vi "Lissajou_Pattern_FOR.vi"() -> ()   [LabVIEW 2019]
panel:
  out "XY Graph":cluster{"X":dbl, "Y":dbl}[](graph)=[{"X"=0.9999996829318346, "Y"=0.0}, {"X"=0.9824361560225692, "Y"=0.12533323356430426}, {"X"=0.9300693384999064, "Y"=0.2486898871648548}, {"X"=0.8447543509816771, "Y"=0.368124552684678}, {"X"=0.7295135194338724, "Y"=0.4817536741017153}, {"X"=0.5884293077665393, "Y"=0.5877852522924731}, {"X"=0.42649969451448655, "Y"=0.6845471059286887}, {"X"=0.2494611169559819, "Y"=0.7705132427757893}, {"X"=0.06358525496231208, "Y"=0.8443279255020151}, {"X"=-0.1245431463883574, "Y"=0.9048270524660195}, {"X"=-0.3082595446881533, "Y"=0.9510565162951535}, {"X"=-0.4810556949368487, "Y"=0.9822872507286886}, {"X"=-0.6368102073656385, "Y"=0.9980267284282716}, {"X"=-0.7700054007214696, "Y"=0.9980267284282716}, {"X"=-0.8759227688762309, "Y"=0.9822872507286887}, {"X"=-0.9508101362587172, "Y"=0.9510565162951536}, {"X"=-0.9920145805448598, "Y"=0.9048270524660195}, {"X"=-0.9980764137536499, "Y"=0.844327925502015}, {"X"=-0.9687808924215839, "Y"=0.7705132427757895}, {"X"=-0.9051658249969167, "Y"=0.6845471059286888}, {"X"=-0.8094848069579887, "Y"=0.5877852522924732}, {"X"=-0.685127386069896, "Y"=0.4817536741017152}, {"X"=-0.5364989859650733, "Y"=0.36812455268467814}, {"X"=-0.36886484181482637, "Y"=0.24868988716485482}, {"X"=-0.18816347674844278, "Y"=0.1253332335643041}, {"X"=-0.000796326710733225, "Y"=1.2246467991473532e-16}, {"X"=0.18659903359770685, "Y"=-0.12533323356430384}, {"X"=0.36738403011337656, "Y"=-0.24868988716485457}, {"X"=0.535154264205682, "Y"=-0.3681245526846779}, {"X"=0.6839663916912916, "Y"=-0.4817536741017154}, {"X"=0.8085486687648371, "Y"=-0.587785252292473}, {"X"=0.9044877061514156, "Y"=-0.6845471059286887}, {"X"=0.9683848156219065, "Y"=-0.7705132427757894}, {"X"=0.9979764102178857, "Y"=-0.8443279255020153}, {"X"=0.9922141929481194, "Y"=-0.9048270524660198}, {"X"=0.9513022932321, "Y"=-0.9510565162951535}, {"X"=0.8766900355135938, "Y"=-0.9822872507286885}, {"X"=0.7710205962196693, "Y"=-0.9980267284282716}, {"X"=0.6380373679180319, "Y"=-0.9980267284282716}, {"X"=0.4824513477690753, "Y"=-0.9822872507286887}, {"X"=0.30977424810283877, "Y"=-0.9510565162951536}, {"X"=0.12612324126189484, "Y"=-0.9048270524660196}, {"X"=-0.06199574427856494, "Y"=-0.844327925502015}, {"X"=-0.24791849967043386, "Y"=-0.7705132427757896}, {"X"=-0.42505861861354033, "Y"=-0.684547105928689}, {"X"=-0.5871408240824221, "Y"=-0.5877852522924734}, {"X"=-0.7284232731434592, "Y"=-0.4817536741017153}, {"X"=-0.8439009646033401, "Y"=-0.36812455268467786}, {"X"=-0.9294830436715473, "Y"=-0.2486898871648545}, {"X"=-0.9821377225307751, "Y"=-0.12533323356430465}, {"X"=-0.9999996829318346, "Y"=-2.4492935982947064e-16}, {"X"=-0.9824361560225694, "Y"=0.1253332335643033}, {"X"=-0.9300693384999066, "Y"=0.24868988716485402}, {"X"=-0.844754350981678, "Y"=0.36812455268467736}, {"X"=-0.729513519433873, "Y"=0.4817536741017149}, {"X"=-0.5884293077665396, "Y"=0.5877852522924729}, {"X"=-0.4264996945144877, "Y"=0.6845471059286886}, {"X"=-0.24946111695598225, "Y"=0.7705132427757893}, {"X"=-0.06358525496231156, "Y"=0.8443279255020152}, {"X"=0.12454314638835703, "Y"=0.9048270524660194}, {"X"=0.3082595446881513, "Y"=0.9510565162951535}, {"X"=0.48105569493684763, "Y"=0.9822872507286886}, {"X"=0.6368102073656382, "Y"=0.9980267284282716}, {"X"=0.7700054007214688, "Y"=0.9980267284282716}, {"X"=0.8759227688762307, "Y"=0.9822872507286886}, {"X"=0.9508101362587175, "Y"=0.9510565162951536}, {"X"=0.9920145805448597, "Y"=0.9048270524660192}, {"X"=0.9980764137536499, "Y"=0.8443279255020151}, {"X"=0.9687808924215838, "Y"=0.7705132427757886}, {"X"=0.9051658249969168, "Y"=0.6845471059286884}, {"X"=0.809484806957989, "Y"=0.5877852522924734}, {"X"=0.6851273860698982, "Y"=0.4817536741017162}, {"X"=0.5364989859650751, "Y"=0.3681245526846796}, {"X"=0.36886484181482754, "Y"=0.2486898871648555}, {"X"=0.18816347674844575, "Y"=0.12533323356430567}, {"X"=0.0007963267107353688, "Y"=3.6739403974420594e-16}, {"X"=-0.1865990335977056, "Y"=-0.12533323356430318}, {"X"=-0.36738403011337295, "Y"=-0.24868988716485477}, {"X"=-0.535154264205681, "Y"=-0.36812455268467725}, {"X"=-0.6839663916912894, "Y"=-0.48175367410171555}, {"X"=-0.8085486687648374, "Y"=-0.5877852522924728}, {"X"=-0.904487706151415, "Y"=-0.6845471059286892}, {"X"=-0.9683848156219059, "Y"=-0.7705132427757891}, {"X"=-0.9979764102178857, "Y"=-0.8443279255020156}, {"X"=-0.9922141929481196, "Y"=-0.9048270524660197}, {"X"=-0.9513022932321007, "Y"=-0.9510565162951534}, {"X"=-0.8766900355135949, "Y"=-0.9822872507286885}, {"X"=-0.7710205962196708, "Y"=-0.9980267284282714}, {"X"=-0.6380373679180322, "Y"=-0.9980267284282716}, {"X"=-0.4824513477690771, "Y"=-0.9822872507286889}, {"X"=-0.3097742481028425, "Y"=-0.9510565162951538}, {"X"=-0.1261232412618952, "Y"=-0.90482705246602}, {"X"=0.061995744278562796, "Y"=-0.8443279255020152}, {"X"=0.24791849967043178, "Y"=-0.7705132427757898}, {"X"=0.42505861861354, "Y"=-0.6845471059286885}, {"X"=0.5871408240824219, "Y"=-0.5877852522924735}, {"X"=0.7284232731434602, "Y"=-0.48175367410171477}, {"X"=0.84390096460334, "Y"=-0.3681245526846781}, {"X"=0.9294830436715465, "Y"=-0.2486898871648556}, {"X"=0.9821377225307754, "Y"=-0.125333233564304}, {"X"=0.9999996829318346, "Y"=-4.898587196589413e-16}, {"X"=0.9824361560225694, "Y"=0.1253332335643048}, {"X"=0.9300693384999074, "Y"=0.24868988716485294}, {"X"=0.8447543509816792, "Y"=0.36812455268467714}, {"X"=0.7295135194338732, "Y"=0.4817536741017139}, {"X"=0.5884293077665413, "Y"=0.5877852522924727}, {"X"=0.42649969451448966, "Y"=0.6845471059286877}, {"X"=0.2494611169559826, "Y"=0.7705132427757891}, {"X"=0.0635852549623137, "Y"=0.8443279255020146}, {"X"=-0.1245431463883549, "Y"=0.9048270524660196}, {"X"=-0.30825954468815264, "Y"=0.9510565162951534}, {"X"=-0.4810556949368473, "Y"=0.9822872507286888}, {"X"=-0.6368102073656365, "Y"=0.9980267284282716}, {"X"=-0.7700054007214697, "Y"=0.9980267284282717}, {"X"=-0.8759227688762306, "Y"=0.9822872507286886}, {"X"=-0.9508101362587168, "Y"=0.9510565162951538}, {"X"=-0.9920145805448598, "Y"=0.9048270524660194}, {"X"=-0.9980764137536499, "Y"=0.8443279255020152}, {"X"=-0.9687808924215844, "Y"=0.7705132427757898}, {"X"=-0.9051658249969177, "Y"=0.6845471059286898}, {"X"=-0.8094848069579913, "Y"=0.5877852522924736}, {"X"=-0.6851273860698972, "Y"=0.48175367410171643}, {"X"=-0.5364989859650754, "Y"=0.3681245526846782}, {"X"=-0.36886484181482954, "Y"=0.2486898871648557}, {"X"=-0.18816347674844436, "Y"=0.12533323356430415}, {"X"=-0.0007963267107357361, "Y"=6.123233995736766e-16}, {"X"=0.1865990335977035, "Y"=-0.12533323356430293}, {"X"=0.3673840301133759, "Y"=-0.24868988716485452}, {"X"=0.5351542642056807, "Y"=-0.3681245526846787}, {"X"=0.683966391691289, "Y"=-0.4817536741017153}, {"X"=0.8085486687648372, "Y"=-0.5877852522924726}, {"X"=0.9044877061514149, "Y"=-0.6845471059286876}, {"X"=0.9683848156219058, "Y"=-0.7705132427757901}, {"X"=0.9979764102178857, "Y"=-0.8443279255020155}, {"X"=0.9922141929481196, "Y"=-0.9048270524660196}, {"X"=0.9513022932321008, "Y"=-0.9510565162951534}, {"X"=0.8766900355135934, "Y"=-0.982287250728689}, {"X"=0.7710205962196687, "Y"=-0.9980267284282717}, {"X"=0.6380373679180324, "Y"=-0.9980267284282716}, {"X"=0.48245134776907433, "Y"=-0.9822872507286887}, {"X"=0.3097742481028395, "Y"=-0.9510565162951538}, {"X"=0.12612324126189908, "Y"=-0.9048270524660201}, {"X"=-0.06199574427855889, "Y"=-0.8443279255020162}, {"X"=-0.24791849967043142, "Y"=-0.770513242775791}, {"X"=-0.42505861861353644, "Y"=-0.6845471059286913}, {"X"=-0.5871408240824186, "Y"=-0.5877852522924737}, {"X"=-0.7284232731434576, "Y"=-0.48175367410171654}, {"X"=-0.8439009646033379, "Y"=-0.36812455268468}, {"X"=-0.9294830436715451, "Y"=-0.24868988716485754}, {"X"=-0.9821377225307747, "Y"=-0.12533323356430426}, {"X"=-0.9999996829318346, "Y"=-7.347880794884119e-16}, {"X"=-0.9824361560225702, "Y"=0.12533323356430282}, {"X"=-0.9300693384999075, "Y"=0.24868988716485269}, {"X"=-0.8447543509816794, "Y"=0.36812455268467525}, {"X"=-0.7295135194338759, "Y"=0.4817536741017152}, {"X"=-0.5884293077665417, "Y"=0.5877852522924725}, {"X"=-0.42649969451448994, "Y"=0.6845471059286876}, {"X"=-0.24946111695598294, "Y"=0.7705132427757878}, {"X"=-0.06358525496231407, "Y"=0.8443279255020154}, {"X"=0.12454314638835454, "Y"=0.9048270524660195}, {"X"=0.3082595446881523, "Y"=0.9510565162951533}, {"X"=0.48105569493684697, "Y"=0.9822872507286884}, {"X"=0.6368102073656363, "Y"=0.9980267284282717}, {"X"=0.7700054007214695, "Y"=0.9980267284282716}, {"X"=0.8759227688762287, "Y"=0.9822872507286887}, {"X"=0.9508101362587167, "Y"=0.9510565162951539}, {"X"=0.9920145805448598, "Y"=0.9048270524660187}, {"X"=0.9980764137536501, "Y"=0.8443279255020144}, {"X"=0.9687808924215844, "Y"=0.7705132427757888}, {"X"=0.9051658249969163, "Y"=0.6845471059286887}, {"X"=0.8094848069579915, "Y"=0.5877852522924738}, {"X"=0.6851273860698974, "Y"=0.4817536741017135}, {"X"=0.5364989859650787, "Y"=0.3681245526846801}, {"X"=0.36886484181482987, "Y"=0.24868988716485768}, {"X"=0.18816347674845169, "Y"=0.12533323356430792}, {"X"=0.0007963267107396562, "Y"=8.572527594031472e-16}, {"X"=-0.18659903359770313, "Y"=-0.12533323356430268}, {"X"=-0.36738403011336895, "Y"=-0.24868988716485257}, {"X"=-0.5351542642056774, "Y"=-0.36812455268467514}, {"X"=-0.6839663916912888, "Y"=-0.4817536741017151}, {"X"=-0.8085486687648329, "Y"=-0.5877852522924725}, {"X"=-0.9044877061514133, "Y"=-0.6845471059286875}, {"X"=-0.9683848156219058, "Y"=-0.7705132427757877}, {"X"=-0.9979764102178853, "Y"=-0.8443279255020134}, {"X"=-0.9922141929481202, "Y"=-0.9048270524660195}, {"X"=-0.9513022932321009, "Y"=-0.9510565162951533}, {"X"=-0.8766900355135969, "Y"=-0.9822872507286884}, {"X"=-0.7710205962196712, "Y"=-0.9980267284282714}, {"X"=-0.6380373679180328, "Y"=-0.9980267284282716}, {"X"=-0.48245134776907467, "Y"=-0.9822872507286887}, {"X"=-0.3097742481028432, "Y"=-0.9510565162951539}, {"X"=-0.12612324126189592, "Y"=-0.9048270524660202}, {"X"=0.061995744278565613, "Y"=-0.8443279255020144}, {"X"=0.24791849967043106, "Y"=-0.7705132427757889}, {"X"=0.42505861861353933, "Y"=-0.6845471059286888}, {"X"=0.5871408240824241, "Y"=-0.5877852522924739}, {"X"=0.7284232731434572, "Y"=-0.4817536741017167}, {"X"=0.8439009646033395, "Y"=-0.36812455268467686}, {"X"=0.9294830436715477, "Y"=-0.24868988716485435}, {"X"=0.9821377225307746, "Y"=-0.1253332335643045}, {"X"=0.9999996829318346, "Y"=-9.797174393178826e-16}, {"X"=0.982436156022569, "Y"=0.1253332335643061}, {"X"=0.9300693384999076, "Y"=0.2486898871648559}, {"X"=0.8447543509816776, "Y"=0.36812455268467836}, {"X"=0.7295135194338761, "Y"=0.4817536741017119}, {"X"=0.5884293077665419, "Y"=0.5877852522924724}, {"X"=0.4264996945144935, "Y"=0.6845471059286874}, {"X"=0.24946111695598674, "Y"=0.7705132427757877}, {"X"=0.06358525496231443, "Y"=0.8443279255020134}, {"X"=-0.12454314638835065, "Y"=0.9048270524660179}, {"X"=-0.30825954468814853, "Y"=0.9510565162951533}, {"X"=-0.48105569493684663, "Y"=0.9822872507286884}, {"X"=-0.6368102073656332, "Y"=0.9980267284282714}, {"X"=-0.770005400721467, "Y"=0.9980267284282718}, {"X"=-0.8759227688762301, "Y"=0.9822872507286887}, {"X"=-0.9508101362587155, "Y"=0.9510565162951539}, {"X"=-0.9920145805448592, "Y"=0.9048270524660202}, {"X"=-0.9980764137536499, "Y"=0.8443279255020164}, {"X"=-0.9687808924215854, "Y"=0.770513242775789}, {"X"=-0.905165824996918, "Y"=0.684547105928689}, {"X"=-0.8094848069579896, "Y"=0.587785252292474}, {"X"=-0.6851273860699003, "Y"=0.4817536741017168}, {"X"=-0.5364989859650761, "Y"=0.368124552684677}, {"X"=-0.3688648418148269, "Y"=0.24868988716485446}, {"X"=-0.18816347674844858, "Y"=0.12533323356430462}, {"X"=-0.0007963267107364708, "Y"=1.102182119232618e-15}, {"X"=0.18659903359770627, "Y"=-0.12533323356430245}, {"X"=0.3673840301133719, "Y"=-0.24868988716485577}, {"X"=0.5351542642056801, "Y"=-0.36812455268467825}, {"X"=0.6839663916912911, "Y"=-0.48175367410171493}, {"X"=0.8085486687648347, "Y"=-0.5877852522924722}, {"X"=0.9044877061514146, "Y"=-0.68454710592869}, {"X"=0.9683848156219066, "Y"=-0.7705132427757898}, {"X"=0.9979764102178855, "Y"=-0.8443279255020152}, {"X"=0.9922141929481197, "Y"=-0.9048270524660194}, {"X"=0.9513022932321021, "Y"=-0.9510565162951532}, {"X"=0.8766900355135954, "Y"=-0.9822872507286883}, {"X"=0.7710205962196737, "Y"=-0.9980267284282714}, {"X"=0.6380373679180358, "Y"=-0.9980267284282718}, {"X"=0.4824513477690781, "Y"=-0.9822872507286894}, {"X"=0.3097742481028469, "Y"=-0.951056516295154}, {"X"=0.1261232412618998, "Y"=-0.9048270524660204}, {"X"=-0.0619957442785617, "Y"=-0.8443279255020165}, {"X"=-0.24791849967042728, "Y"=-0.7705132427757914}, {"X"=-0.4250586186135358, "Y"=-0.684547105928689}, {"X"=-0.587140824082421, "Y"=-0.5877852522924741}, {"X"=-0.7284232731434546, "Y"=-0.48175367410171693}, {"X"=-0.8439009646033374, "Y"=-0.3681245526846804}, {"X"=-0.9294830436715461, "Y"=-0.2486898871648546}, {"X"=-0.9821377225307738, "Y"=-0.12533323356430476}, {"X"=-0.9999996829318346, "Y"=-1.2246467991473533e-15}, {"X"=-0.9824361560225696, "Y"=0.12533323356430232}, {"X"=-0.930069338499909, "Y"=0.2486898871648522}, {"X"=-0.8447543509816797, "Y"=0.36812455268467814}, {"X"=-0.729513519433874, "Y"=0.4817536741017148}, {"X"=-0.5884293077665451, "Y"=0.587785252292475}, {"X"=-0.4264996945144906, "Y"=0.6845471059286898}, {"X"=-0.24946111695598366, "Y"=0.7705132427757898}, {"X"=-0.06358525496231834, "Y"=0.8443279255020152}, {"X"=0.12454314638835381, "Y"=0.9048270524660192}, {"X"=0.3082595446881516, "Y"=0.9510565162951532}, {"X"=0.4810556949368432, "Y"=0.9822872507286883}, {"X"=0.6368102073656356, "Y"=0.9980267284282713}, {"X"=0.7700054007214691, "Y"=0.9980267284282713}, {"X"=0.8759227688762283, "Y"=0.9822872507286882}, {"X"=0.9508101362587165, "Y"=0.9510565162951529}, {"X"=0.9920145805448597, "Y"=0.9048270524660189}, {"X"=0.9980764137536502, "Y"=0.8443279255020146}, {"X"=0.9687808924215846, "Y"=0.7705132427757891}, {"X"=0.9051658249969167, "Y"=0.6845471059286891}, {"X"=0.809484806957992, "Y"=0.5877852522924742}, {"X"=0.685127386069898, "Y"=0.48175367410171704}, {"X"=0.5364989859650733, "Y"=0.3681245526846739}, {"X"=0.36886484181483054, "Y"=0.24868988716485127}, {"X"=0.18816347674844544, "Y"=0.12533323356430134}, {"X"=0.0007963267107332856, "Y"=-2.2056021997384123e-15}, {"X"=-0.1865990335977024, "Y"=-0.12533323356430573}, {"X"=-0.3673840301133749, "Y"=-0.24868988716485554}, {"X"=-0.5351542642056828, "Y"=-0.36812455268467803}, {"X"=-0.6839663916912883, "Y"=-0.4817536741017147}, {"X"=-0.8085486687648366, "Y"=-0.587785252292472}, {"X"=-0.9044877061514159, "Y"=-0.6845471059286923}, {"X"=-0.9683848156219038, "Y"=-0.7705132427757875}, {"X"=-0.9979764102178852, "Y"=-0.8443279255020132}, {"X"=-0.9922141929481211, "Y"=-0.9048270524660177}, {"X"=-0.9513022932321034, "Y"=-0.9510565162951521}, {"X"=-0.8766900355135973, "Y"=-0.9822872507286876}, {"X"=-0.7710205962196762, "Y"=-0.9980267284282711}, {"X"=-0.6380373679180388, "Y"=-0.998026728428272}, {"X"=-0.48245134776908155, "Y"=-0.9822872507286888}, {"X"=-0.30977424810285065, "Y"=-0.951056516295154}, {"X"=-0.1261232412619037, "Y"=-0.9048270524660205}, {"X"=0.061995744278557786, "Y"=-0.8443279255020166}, {"X"=0.24791849967042348, "Y"=-0.7705132427757915}, {"X"=0.4250586186135322, "Y"=-0.6845471059286918}, {"X"=0.5871408240824177, "Y"=-0.5877852522924771}, {"X"=0.7284232731434519, "Y"=-0.48175367410172026}, {"X"=0.8439009646033353, "Y"=-0.3681245526846839}, {"X"=0.9294830436715447, "Y"=-0.24868988716485482}, {"X"=0.9821377225307731, "Y"=-0.12533323356430498}, {"X"=0.9999996829318346, "Y"=-1.4695761589768238e-15}, {"X"=0.9824361560225704, "Y"=0.12533323356430207}, {"X"=0.9300693384999105, "Y"=0.248689887164852}, {"X"=0.8447543509816818, "Y"=0.3681245526846746}, {"X"=0.7295135194338767, "Y"=0.4817536741017115}, {"X"=0.5884293077665482, "Y"=0.587785252292469}, {"X"=0.42649969451449415, "Y"=0.6845471059286845}, {"X"=0.24946111695598747, "Y"=0.7705132427757896}, {"X"=0.06358525496232226, "Y"=0.8443279255020151}, {"X"=-0.12454314638834992, "Y"=0.9048270524660192}, {"X"=-0.30825954468814787, "Y"=0.9510565162951531}, {"X"=-0.48105569493683975, "Y"=0.9822872507286883}, {"X"=-0.6368102073656327, "Y"=0.9980267284282713}, {"X"=-0.7700054007214665, "Y"=0.9980267284282718}, {"X"=-0.8759227688762298, "Y"=0.9822872507286895}, {"X"=-0.9508101362587152, "Y"=0.951056516295153}, {"X"=-0.9920145805448591, "Y"=0.904827052466019}, {"X"=-0.99807641375365, "Y"=0.8443279255020147}, {"X"=-0.9687808924215856, "Y"=0.7705132427757894}, {"X"=-0.9051658249969183, "Y"=0.6845471059286893}, {"X"=-0.8094848069579901, "Y"=0.5877852522924744}, {"X"=-0.6851273860699008, "Y"=0.48175367410171727}, {"X"=-0.5364989859650766, "Y"=0.36812455268468075}, {"X"=-0.3688648418148276, "Y"=0.24868988716485838}, {"X"=-0.1881634767484493, "Y"=0.1253332335643016}, {"X"=-0.0007963267107372057, "Y"=-1.9606728399089416e-15}, {"X"=0.18659903359770555, "Y"=-0.12533323356430548}, {"X"=0.36738403011337123, "Y"=-0.2486898871648553}, {"X"=0.5351542642056795, "Y"=-0.3681245526846778}, {"X"=0.6839663916912906, "Y"=-0.4817536741017145}, {"X"=0.8085486687648342, "Y"=-0.5877852522924718}, {"X"=0.9044877061514143, "Y"=-0.684547105928687}, {"X"=0.9683848156219046, "Y"=-0.7705132427757918}, {"X"=0.997976410217885, "Y"=-0.8443279255020169}, {"X"=0.9922141929481199, "Y"=-0.9048270524660207}, {"X"=0.9513022932321024, "Y"=-0.9510565162951542}, {"X"=0.8766900355135991, "Y"=-0.9822872507286889}, {"X"=0.7710205962196697, "Y"=-0.9980267284282716}, {"X"=0.6380373679180363, "Y"=-0.9980267284282716}, {"X"=0.482451347769085, "Y"=-0.9822872507286888}, {"X"=0.30977424810285437, "Y"=-0.9510565162951541}, {"X"=0.12612324126190053, "Y"=-0.9048270524660175}, {"X"=-0.06199574427855387, "Y"=-0.844327925502013}, {"X"=-0.24791849967041968, "Y"=-0.7705132427757871}, {"X"=-0.4250586186135223, "Y"=-0.684547105928692}, {"X"=-0.5871408240824031, "Y"=-0.5877852522924774}, {"X"=-0.7284232731434492, "Y"=-0.4817536741017205}, {"X"=-0.8439009646033294, "Y"=-0.3681245526846842}, {"X"=-0.929483043671538, "Y"=-0.24868988716486196}, {"X"=-0.9821377225307724, "Y"=-0.12533323356431228}, {"X"=-0.9999996829318346, "Y"=-1.7145055188062944e-15}, {"X"=-0.9824361560225737, "Y"=0.12533323356430184}, {"X"=-0.9300693384999119, "Y"=0.24868988716485174}, {"X"=-0.8447543509816877, "Y"=0.36812455268467437}, {"X"=-0.7295135194338891, "Y"=0.48175367410171127}, {"X"=-0.5884293077665514, "Y"=0.5877852522924688}, {"X"=-0.42649969451450415, "Y"=0.6845471059286843}, {"X"=-0.249461116956005, "Y"=0.7705132427757849}, {"X"=-0.06358525496232617, "Y"=0.8443279255020149}, {"X"=0.12454314638833898, "Y"=0.9048270524660191}, {"X"=0.3082595446881306, "Y"=0.951056516295153}, {"X"=0.4810556949368363, "Y"=0.9822872507286882}, {"X"=0.6368102073656242, "Y"=0.9980267284282713}, {"X"=0.770005400721455, "Y"=0.9980267284282718}, {"X"=0.8759227688762244, "Y"=0.9822872507286895}, {"X"=0.9508101362587118, "Y"=0.9510565162951552}, {"X"=0.9920145805448569, "Y"=0.9048270524660221}, {"X"=0.9980764137536506, "Y"=0.8443279255020149}, {"X"=0.9687808924215883, "Y"=0.7705132427757895}, {"X"=0.905165824996926, "Y"=0.6845471059286894}, {"X"=0.8094848069579966, "Y"=0.5877852522924746}, {"X"=0.6851273860699089, "Y"=0.4817536741017175}, {"X"=0.5364989859650919, "Y"=0.368124552684681}, {"X"=0.36886484181483786, "Y"=0.24868988716485863}, {"X"=0.18816347674846012, "Y"=0.1253332335643089}, {"X"=0.0007963267107553366, "Y"=5.3896838775215305e-15}, {"X"=-0.18659903359769472, "Y"=-0.12533323356430523}, {"X"=-0.36738403011336096, "Y"=-0.24868988716485507}, {"X"=-0.5351542642056761, "Y"=-0.3681245526846776}, {"X"=-0.6839663916912826, "Y"=-0.48175367410171427}, {"X"=-0.8085486687648278, "Y"=-0.5877852522924716}, {"X"=-0.9044877061514126, "Y"=-0.6845471059286867}, {"X"=-0.9683848156219036, "Y"=-0.7705132427757871}, {"X"=-0.9979764102178847, "Y"=-0.844327925502013}, {"X"=-0.9922141929481203, "Y"=-0.9048270524660206}, {"X"=-0.9513022932321036, "Y"=-0.9510565162951541}, {"X"=-0.876690035513601, "Y"=-0.9822872507286888}, {"X"=-0.7710205962196721, "Y"=-0.9980267284282716}, {"X"=-0.6380373679180393, "Y"=-0.9980267284282716}, {"X"=-0.4824513477690884, "Y"=-0.9822872507286889}, {"X"=-0.3097742481028446, "Y"=-0.9510565162951542}, {"X"=-0.12612324126190444, "Y"=-0.9048270524660207}, {"X"=0.06199574427854996, "Y"=-0.8443279255020169}, {"X"=0.24791849967042964, "Y"=-0.7705132427757873}, {"X"=0.42505861861353156, "Y"=-0.684547105928687}, {"X"=0.5871408240824114, "Y"=-0.5877852522924718}, {"X"=0.7284232731434562, "Y"=-0.4817536741017145}, {"X"=0.843900964603335, "Y"=-0.3681245526846778}, {"X"=0.9294830436715418, "Y"=-0.2486898871648553}, {"X"=0.9821377225307744, "Y"=-0.12533323356430548}, {"X"=0.9999996829318346, "Y"=-1.959434878635765e-15}, {"X"=0.9824361560225718, "Y"=0.12533323356430864}, {"X"=0.9300693384999081, "Y"=0.24868988716485838}, {"X"=0.8447543509816822, "Y"=0.36812455268468075}, {"X"=0.729513519433882, "Y"=0.48175367410171727}, {"X"=0.5884293077665431, "Y"=0.5877852522924744}, {"X"=0.4264996945144948, "Y"=0.6845471059286893}, {"X"=0.24946111695599504, "Y"=0.7705132427757848}, {"X"=0.06358525496233008, "Y"=0.844327925502011}, {"X"=-0.1245431463883351, "Y"=0.9048270524660159}, {"X"=-0.3082595446881404, "Y"=0.951056516295153}, {"X"=-0.4810556949368329, "Y"=0.9822872507286882}, {"X"=-0.6368102073656211, "Y"=0.9980267284282713}, {"X"=-0.7700054007214615, "Y"=0.9980267284282718}, {"X"=-0.8759227688762226, "Y"=0.9822872507286896}, {"X"=-0.9508101362587106, "Y"=0.9510565162951553}, {"X"=-0.9920145805448582, "Y"=0.9048270524660222}, {"X"=-0.9980764137536509, "Y"=0.8443279255020189}, {"X"=-0.9687808924215893, "Y"=0.7705132427757941}, {"X"=-0.9051658249969217, "Y"=0.6845471059286896}, {"X"=-0.8094848069579988, "Y"=0.5877852522924748}, {"X"=-0.6851273860699117, "Y"=0.4817536741017177}, {"X"=-0.5364989859650833, "Y"=0.3681245526846812}, {"X"=-0.36886484181484147, "Y"=0.24868988716485885}, {"X"=-0.18816347674846398, "Y"=0.12533323356430912}, {"X"=-0.0007963267107450459, "Y"=5.6346132373510016e-15}, {"X"=0.18659903359769087, "Y"=-0.12533323356429796}, {"X"=0.3673840301133573, "Y"=-0.24868988716485482}, {"X"=0.5351542642056728, "Y"=-0.3681245526846773}, {"X"=0.6839663916912797, "Y"=-0.48175367410171405}, {"X"=0.8085486687648255, "Y"=-0.5877852522924714}, {"X"=0.9044877061514109, "Y"=-0.6845471059286866}, {"X"=0.9683848156219027, "Y"=-0.770513242775787}, {"X"=0.9979764102178845, "Y"=-0.8443279255020129}, {"X"=0.9922141929481209, "Y"=-0.9048270524660175}, {"X"=0.9513022932321048, "Y"=-0.9510565162951519}, {"X"=0.8766900355136029, "Y"=-0.9822872507286888}, {"X"=0.7710205962196747, "Y"=-0.9980267284282716}, {"X"=0.6380373679180424, "Y"=-0.9980267284282716}, {"X"=0.4824513477690918, "Y"=-0.9822872507286889}, {"X"=0.3097742481028483, "Y"=-0.9510565162951542}, {"X"=0.12612324126190833, "Y"=-0.9048270524660208}, {"X"=-0.06199574427854605, "Y"=-0.844327925502017}, {"X"=-0.24791849967042584, "Y"=-0.7705132427757919}, {"X"=-0.425058618613528, "Y"=-0.6845471059286872}, {"X"=-0.5871408240824082, "Y"=-0.587785252292472}, {"X"=-0.7284232731434536, "Y"=-0.4817536741017147}, {"X"=-0.8439009646033329, "Y"=-0.36812455268467803}, {"X"=-0.9294830436715403, "Y"=-0.24868988716485554}, {"X"=-0.9821377225307736, "Y"=-0.12533323356430573}, {"X"=-0.9999996829318346, "Y"=-2.204364238465236e-15}, {"X"=-0.9824361560225726, "Y"=0.12533323356430134}, {"X"=-0.9300693384999096, "Y"=0.24868988716485127}, {"X"=-0.8447543509816843, "Y"=0.36812455268468053}, {"X"=-0.7295135194338848, "Y"=0.48175367410171704}, {"X"=-0.5884293077665463, "Y"=0.5877852522924742}, {"X"=-0.4264996945144984, "Y"=0.6845471059286891}, {"X"=-0.24946111695599885, "Y"=0.7705132427757891}, {"X"=-0.06358525496231981, "Y"=0.8443279255020146}, {"X"=0.12454314638834531, "Y"=0.9048270524660189}, {"X"=0.30825954468813666, "Y"=0.9510565162951529}, {"X"=0.4810556949368419, "Y"=0.9822872507286882}, {"X"=0.6368102073656291, "Y"=0.9980267284282718}, {"X"=0.7700054007214591, "Y"=0.9980267284282713}, {"X"=0.8759227688762276, "Y"=0.9822872507286883}, {"X"=0.9508101362587138, "Y"=0.9510565162951532}, {"X"=0.9920145805448577, "Y"=0.9048270524660192}, {"X"=0.9980764137536502, "Y"=0.8443279255020152}, {"X"=0.9687808924215867, "Y"=0.7705132427757898}, {"X"=0.9051658249969233, "Y"=0.6845471059286949}, {"X"=0.8094848069580012, "Y"=0.587785252292475}, {"X"=0.6851273860699145, "Y"=0.48175367410171793}, {"X"=0.5364989859650866, "Y"=0.3681245526846814}, {"X"=0.36886484181484513, "Y"=0.2486898871648591}, {"X"=0.1881634767484678, "Y"=0.12533323356430937}, {"X"=0.000796326710748966, "Y"=5.879542597180472e-15}, {"X"=-0.186599033597687, "Y"=-0.1253332335642977}, {"X"=-0.3673840301133537, "Y"=-0.24868988716484772}, {"X"=-0.5351542642056695, "Y"=-0.3681245526846705}, {"X"=-0.6839663916912768, "Y"=-0.4817536741017138}, {"X"=-0.8085486687648232, "Y"=-0.5877852522924712}, {"X"=-0.9044877061514093, "Y"=-0.6845471059286864}, {"X"=-0.9683848156219017, "Y"=-0.7705132427757868}, {"X"=-0.9979764102178842, "Y"=-0.8443279255020126}, {"X"=-0.9922141929481213, "Y"=-0.9048270524660174}, {"X"=-0.951302293232106, "Y"=-0.9510565162951518}, {"X"=-0.8766900355136048, "Y"=-0.9822872507286874}, {"X"=-0.7710205962196771, "Y"=-0.9980267284282711}, {"X"=-0.6380373679180454, "Y"=-0.9980267284282717}, {"X"=-0.48245134776909526, "Y"=-0.9822872507286889}, {"X"=-0.30977424810285203, "Y"=-0.9510565162951543}, {"X"=-0.1261232412619122, "Y"=-0.9048270524660209}, {"X"=0.06199574427854214, "Y"=-0.8443279255020172}, {"X"=0.24791849967042207, "Y"=-0.7705132427757921}, {"X"=0.4250586186135245, "Y"=-0.6845471059286925}, {"X"=0.5871408240824051, "Y"=-0.587785252292478}, {"X"=0.7284232731434509, "Y"=-0.48175367410171493}, {"X"=0.8439009646033307, "Y"=-0.36812455268467825}, {"X"=0.9294830436715389, "Y"=-0.24868988716485577}, {"X"=0.9821377225307728, "Y"=-0.12533323356430598}, {"X"=0.9999996829318346, "Y"=-2.4492935982947065e-15}, {"X"=0.9824361560225733, "Y"=0.1253332335643011}, {"X"=0.930069338499911, "Y"=0.24868988716485102}, {"X"=0.8447543509816864, "Y"=0.3681245526846737}, {"X"=0.7295135194338874, "Y"=0.4817536741017106}, {"X"=0.5884293077665494, "Y"=0.587785252292474}, {"X"=0.4264996945145019, "Y"=0.684547105928689}, {"X"=0.24946111695600265, "Y"=0.770513242775789}, {"X"=0.06358525496232373, "Y"=0.8443279255020145}, {"X"=-0.12454314638834141, "Y"=0.9048270524660188}, {"X"=-0.30825954468813294, "Y"=0.951056516295155}, {"X"=-0.4810556949368385, "Y"=0.982287250728688}, {"X"=-0.6368102073656261, "Y"=0.9980267284282718}, {"X"=-0.7700054007214565, "Y"=0.9980267284282719}, {"X"=-0.8759227688762257, "Y"=0.9822872507286884}, {"X"=-0.9508101362587126, "Y"=0.9510565162951554}, {"X"=-0.9920145805448572, "Y"=0.9048270524660194}, {"X"=-0.9980764137536505, "Y"=0.8443279255020191}, {"X"=-0.9687808924215877, "Y"=0.7705132427757899}, {"X"=-0.905165824996925, "Y"=0.6845471059286848}, {"X"=-0.8094848069579951, "Y"=0.5877852522924751}, {"X"=-0.6851273860699071, "Y"=0.4817536741017119}, {"X"=-0.5364989859650898, "Y"=0.36812455268468164}, {"X"=-0.3688648418148356, "Y"=0.24868988716485246}, {"X"=-0.1881634767484577, "Y"=0.12533323356430962}, {"X"=-0.0007963267107528861, "Y"=-9.809554005910593e-16}, {"X"=0.18659903359769714, "Y"=-0.12533323356431156}, {"X"=0.36738403011336324, "Y"=-0.24868988716485435}, {"X"=0.5351542642056663, "Y"=-0.36812455268468347}, {"X"=0.6839663916912844, "Y"=-0.4817536741017136}, {"X"=0.8085486687648292, "Y"=-0.5877852522924768}, {"X"=0.9044877061514076, "Y"=-0.6845471059286863}, {"X"=0.9683848156219043, "Y"=-0.7705132427757913}, {"X"=0.9979764102178849, "Y"=-0.8443279255020125}, {"X"=0.9922141929481217, "Y"=-0.9048270524660202}, {"X"=0.9513022932321028, "Y"=-0.9510565162951561}, {"X"=0.8766900355135999, "Y"=-0.9822872507286887}, {"X"=0.7710205962196797, "Y"=-0.998026728428272}, {"X"=0.6380373679180374, "Y"=-0.9980267284282717}, {"X"=0.48245134776908627, "Y"=-0.9822872507286877}, {"X"=0.30977424810285575, "Y"=-0.9510565162951544}, {"X"=0.126123241261902, "Y"=-0.9048270524660179}, {"X"=-0.06199574427855241, "Y"=-0.8443279255020173}, {"X"=-0.24791849967041826, "Y"=-0.7705132427757877}, {"X"=-0.4250586186135338, "Y"=-0.6845471059286823}, {"X"=-0.5871408240824134, "Y"=-0.5877852522924725}, {"X"=-0.7284232731434482, "Y"=-0.4817536741017089}, {"X"=-0.8439009646033363, "Y"=-0.3681245526846785}, {"X"=-0.9294830436715428, "Y"=-0.24868988716484913}, {"X"=-0.9821377225307721, "Y"=-0.1253332335643062}, {"X"=-0.9999996829318346, "Y"=4.411204399476825e-15}, {"X"=-0.9824361560225714, "Y"=0.12533323356430087}, {"X"=-0.9300693384999125, "Y"=0.24868988716485768}, {"X"=-0.844754350981681, "Y"=0.3681245526846867}, {"X"=-0.7295135194338803, "Y"=0.48175367410171666}, {"X"=-0.5884293077665527, "Y"=0.5877852522924796}, {"X"=-0.4264996945144926, "Y"=0.6845471059286887}, {"X"=-0.24946111695599268, "Y"=0.7705132427757934}, {"X"=-0.06358525496232764, "Y"=0.8443279255020144}, {"X"=0.12454314638835162, "Y"=0.9048270524660217}, {"X"=0.3082595446881427, "Y"=0.9510565162951528}, {"X"=0.48105569493683503, "Y"=0.9822872507286894}, {"X"=0.636810207365634, "Y"=0.9980267284282722}, {"X"=0.7700054007214541, "Y"=0.9980267284282723}, {"X"=0.8759227688762169, "Y"=0.9822872507286897}, {"X"=0.9508101362587069, "Y"=0.9510565162951578}, {"X"=0.9920145805448567, "Y"=0.9048270524660226}, {"X"=0.9980764137536516, "Y"=0.8443279255020231}, {"X"=0.9687808924215922, "Y"=0.7705132427757946}, {"X"=0.9051658249969267, "Y"=0.6845471059286902}, {"X"=0.8094848069580057, "Y"=0.5877852522924811}, {"X"=0.6851273860699203, "Y"=0.4817536741017183}, {"X"=0.5364989859650932, "Y"=0.36812455268468847}, {"X"=0.3688648418148524, "Y"=0.24868988716485957}, {"X"=0.18816347674847553, "Y"=0.12533323356431691}, {"X"=0.0007963267107568063, "Y"=6.369401316839413e-15}, {"X"=-0.18659903359767932, "Y"=-0.12533323356429016}, {"X"=-0.36738403011334636, "Y"=-0.24868988716484725}, {"X"=-0.5351542642056629, "Y"=-0.36812455268467664}, {"X"=-0.6839663916912712, "Y"=-0.48175367410170716}, {"X"=-0.8085486687648186, "Y"=-0.5877852522924708}, {"X"=-0.904487706151406, "Y"=-0.6845471059286808}, {"X"=-0.9683848156218997, "Y"=-0.7705132427757865}, {"X"=-0.9979764102178837, "Y"=-0.8443279255020086}, {"X"=-0.9922141929481223, "Y"=-0.9048270524660171}, {"X"=-0.9513022932321085, "Y"=-0.9510565162951494}, {"X"=-0.8766900355136086, "Y"=-0.9822872507286874}, {"X"=-0.7710205962196821, "Y"=-0.9980267284282716}, {"X"=-0.6380373679180514, "Y"=-0.9980267284282721}, {"X"=-0.48245134776910215, "Y"=-0.982287250728689}, {"X"=-0.30977424810285953, "Y"=-0.9510565162951566}, {"X"=-0.12612324126191998, "Y"=-0.904827052466021}, {"X"=0.06199574427853431, "Y"=-0.8443279255020212}, {"X"=0.24791849967041446, "Y"=-0.7705132427757925}, {"X"=0.4250586186135174, "Y"=-0.684547105928698}, {"X"=0.5871408240823988, "Y"=-0.5877852522924784}, {"X"=0.7284232731434455, "Y"=-0.4817536741017153}, {"X"=0.8439009646033265, "Y"=-0.3681245526846853}, {"X"=0.929483043671536, "Y"=-0.24868988716485624}, {"X"=0.9821377225307714, "Y"=-0.1253332335643135}, {"X"=0.9999996829318346, "Y"=-2.9391523179536475e-15}, {"X"=0.9824361560225747, "Y"=0.12533323356429357}, {"X"=0.9300693384999139, "Y"=0.24868988716485055}, {"X"=0.8447543509816906, "Y"=0.36812455268466665}, {"X"=0.7295135194338928, "Y"=0.4817536741017102}, {"X"=0.5884293077665558, "Y"=0.5877852522924736}, {"X"=0.42649969451450903, "Y"=0.6845471059286834}, {"X"=0.24946111695601023, "Y"=0.7705132427757887}, {"X"=0.06358525496233154, "Y"=0.8443279255020104}, {"X"=-0.12454314638833364, "Y"=0.9048270524660186}, {"X"=-0.3082595446881255, "Y"=0.9510565162951504}, {"X"=-0.4810556949368316, "Y"=0.9822872507286879}, {"X"=-0.63681020736562, "Y"=0.9980267284282709}, {"X"=-0.7700054007214515, "Y"=0.9980267284282719}, {"X"=-0.8759227688762219, "Y"=0.9822872507286885}, {"X"=-0.9508101362587101, "Y"=0.9510565162951556}, {"X"=-0.9920145805448563, "Y"=0.9048270524660196}, {"X"=-0.998076413753651, "Y"=0.8443279255020194}, {"X"=-0.9687808924215896, "Y"=0.7705132427757903}, {"X"=-0.9051658249969283, "Y"=0.6845471059286955}, {"X"=-0.8094848069579997, "Y"=0.5877852522924756}, {"X"=-0.6851273860699127, "Y"=0.4817536741017123}, {"X"=-0.5364989859650965, "Y"=0.36812455268468214}, {"X"=-0.36886484181484286, "Y"=0.24868988716485294}, {"X"=-0.18816347674846542, "Y"=0.1253332335643101}, {"X"=-0.0007963267107465154, "Y"=-4.91096680932118e-16}, {"X"=0.18659903359768942, "Y"=-0.125333233564297}, {"X"=0.36738403011335596, "Y"=-0.24868988716485388}, {"X"=0.5351542642056716, "Y"=-0.3681245526846698}, {"X"=0.6839663916912786, "Y"=-0.4817536741017132}, {"X"=0.8085486687648247, "Y"=-0.5877852522924764}, {"X"=0.9044877061514103, "Y"=-0.6845471059286858}, {"X"=0.9683848156219023, "Y"=-0.7705132427757909}, {"X"=0.9979764102178844, "Y"=-0.8443279255020123}, {"X"=0.992214192948121, "Y"=-0.90482705246602}, {"X"=0.9513022932321052, "Y"=-0.9510565162951515}, {"X"=0.8766900355136037, "Y"=-0.9822872507286886}, {"X"=0.7710205962196756, "Y"=-0.998026728428271}, {"X"=0.6380373679180436, "Y"=-0.9980267284282717}, {"X"=0.4824513477690931, "Y"=-0.9822872507286878}, {"X"=0.3097742481028497, "Y"=-0.9510565162951545}, {"X"=0.12612324126190977, "Y"=-0.9048270524660181}, {"X"=-0.06199574427854458, "Y"=-0.8443279255020175}, {"X"=-0.24791849967042442, "Y"=-0.770513242775788}, {"X"=-0.42505861861352673, "Y"=-0.6845471059286931}, {"X"=-0.587140824082407, "Y"=-0.5877852522924728}, {"X"=-0.7284232731434526, "Y"=-0.48175367410172176}, {"X"=-0.8439009646033321, "Y"=-0.3681245526846789}, {"X"=-0.9294830436715398, "Y"=-0.2486898871648496}, {"X"=-0.9821377225307732, "Y"=-0.1253332335643067}, {"X"=-0.9999996829318346, "Y"=3.921345679817883e-15}, {"X"=-0.9824361560225728, "Y"=0.12533323356430037}, {"X"=-0.9300693384999101, "Y"=0.2486898871648572}, {"X"=-0.844754350981685, "Y"=0.368124552684673}, {"X"=-0.7295135194338858, "Y"=0.4817536741017162}, {"X"=-0.5884293077665474, "Y"=0.5877852522924677}, {"X"=-0.4264996945144997, "Y"=0.6845471059286884}, {"X"=-0.24946111695600026, "Y"=0.770513242775793}, {"X"=-0.06358525496232127, "Y"=0.8443279255020141}, {"X"=0.12454314638834385, "Y"=0.9048270524660215}, {"X"=0.30825954468813527, "Y"=0.9510565162951525}, {"X"=0.48105569493684064, "Y"=0.9822872507286893}, {"X"=0.636810207365628, "Y"=0.9980267284282712}, {"X"=0.7700054007214581, "Y"=0.9980267284282714}, {"X"=0.8759227688762269, "Y"=0.9822872507286872}, {"X"=0.9508101362587132, "Y"=0.9510565162951535}, {"X"=0.9920145805448575, "Y"=0.9048270524660167}, {"X"=0.9980764137536503, "Y"=0.8443279255020156}, {"X"=0.968780892421587, "Y"=0.7705132427757859}, {"X"=0.905165824996924, "Y"=0.6845471059286905}, {"X"=0.8094848069579936, "Y"=0.58778525229247}, {"X"=0.685127386069895, "Y"=0.48175367410171877}, {"X"=0.5364989859650878, "Y"=0.36812455268467575}, {"X"=0.3688648418148333, "Y"=0.24868988716484627}, {"X"=0.18816347674844136, "Y"=0.1253332335643033}, {"X"=0.0007963267107504356, "Y"=-7.351594678703649e-15}, {"X"=-0.18659903359769953, "Y"=-0.1253332335643038}, {"X"=-0.3673840301133787, "Y"=-0.2486898871648605}, {"X"=-0.5351542642056683, "Y"=-0.3681245526846762}, {"X"=-0.6839663916912861, "Y"=-0.4817536741017192}, {"X"=-0.8085486687648223, "Y"=-0.5877852522924705}, {"X"=-0.9044877061514086, "Y"=-0.684547105928691}, {"X"=-0.9683848156219048, "Y"=-0.7705132427757952}, {"X"=-0.9979764102178841, "Y"=-0.844327925502016}, {"X"=-0.9922141929481215, "Y"=-0.9048270524660229}, {"X"=-0.9513022932321021, "Y"=-0.9510565162951536}, {"X"=-0.8766900355136056, "Y"=-0.9822872507286899}, {"X"=-0.7710205962196781, "Y"=-0.9980267284282714}, {"X"=-0.6380373679180574, "Y"=-0.9980267284282721}, {"X"=-0.48245134776909654, "Y"=-0.9822872507286918}, {"X"=-0.30977424810288046, "Y"=-0.9510565162951569}, {"X"=-0.12612324126192775, "Y"=-0.9048270524660212}, {"X"=0.06199574427854067, "Y"=-0.8443279255020215}, {"X"=0.2479184996703931, "Y"=-0.7705132427757928}, {"X"=0.4250586186135103, "Y"=-0.6845471059286984}, {"X"=0.5871408240824039, "Y"=-0.5877852522924788}, {"X"=0.7284232731434305, "Y"=-0.4817536741017282}, {"X"=0.8439009646033223, "Y"=-0.36812455268468575}, {"X"=0.9294830436715383, "Y"=-0.24868988716487048}, {"X"=0.9821377225307673, "Y"=-0.125333233564314}, {"X"=0.9999996829318346, "Y"=-3.429011037612589e-15}, {"X"=0.9824361560225736, "Y"=0.12533323356429307}, {"X"=0.930069338499922, "Y"=0.24868988716485008}, {"X"=0.8447543509816948, "Y"=0.36812455268466615}, {"X"=0.7295135194338884, "Y"=0.4817536741017098}, {"X"=0.5884293077665737, "Y"=0.5877852522924617}, {"X"=0.42649969451451614, "Y"=0.6845471059286831}, {"X"=0.24946111695600406, "Y"=0.7705132427757884}, {"X"=0.06358525496235355, "Y"=0.8443279255020102}, {"X"=-0.12454314638832585, "Y"=0.9048270524660184}, {"X"=-0.30825954468813155, "Y"=0.9510565162951503}, {"X"=-0.4810556949368123, "Y"=0.9822872507286879}, {"X"=-0.636810207365614, "Y"=0.9980267284282708}, {"X"=-0.7700054007214556, "Y"=0.9980267284282719}, {"X"=-0.8759227688762112, "Y"=0.9822872507286912}, {"X"=-0.9508101362587077, "Y"=0.9510565162951558}, {"X"=-0.992014580544857, "Y"=0.9048270524660198}, {"X"=-0.9980764137536523, "Y"=0.8443279255020196}, {"X"=-0.9687808924215916, "Y"=0.7705132427757906}, {"X"=-0.9051658249969257, "Y"=0.6845471059286958}, {"X"=-0.8094848069580127, "Y"=0.587785252292476}, {"X"=-0.6851273860699185, "Y"=0.4817536741017252}, {"X"=-0.5364989859650912, "Y"=0.3681245526846826}, {"X"=-0.36886484181486334, "Y"=0.24868988716486717}, {"X"=-0.1881634767484731, "Y"=0.1253332335643106}, {"X"=-0.0007963267107543557, "Y"=-1.2379612731767154e-18}, {"X"=0.18659903359766777, "Y"=-0.1253332335642965}, {"X"=0.36738403011334864, "Y"=-0.2486898871648534}, {"X"=0.5351542642056649, "Y"=-0.36812455268466937}, {"X"=0.6839663916912626, "Y"=-0.48175367410171277}, {"X"=0.80854866876482, "Y"=-0.5877852522924645}, {"X"=0.904487706151407, "Y"=-0.6845471059286855}, {"X"=0.9683848156218968, "Y"=-0.7705132427757815}, {"X"=0.9979764102178839, "Y"=-0.844327925502012}, {"X"=0.992214192948122, "Y"=-0.9048270524660198}, {"X"=0.951302293232112, "Y"=-0.9510565162951513}, {"X"=0.8766900355136075, "Y"=-0.9822872507286885}, {"X"=0.7710205962196806, "Y"=-0.998026728428271}, {"X"=0.6380373679180605, "Y"=-0.9980267284282717}, {"X"=0.4824513477691, "Y"=-0.9822872507286906}, {"X"=0.3097742481028572, "Y"=-0.9510565162951546}, {"X"=0.12612324126193164, "Y"=-0.9048270524660245}, {"X"=-0.061995744278536755, "Y"=-0.8443279255020179}, {"X"=-0.24791849967041682, "Y"=-0.7705132427757884}, {"X"=-0.42505861861350674, "Y"=-0.6845471059286934}, {"X"=-0.5871408240824006, "Y"=-0.5877852522924732}, {"X"=-0.7284232731434471, "Y"=-0.4817536741017222}, {"X"=-0.8439009646033202, "Y"=-0.36812455268467936}, {"X"=-0.9294830436715369, "Y"=-0.24868988716486384}, {"X"=-0.9821377225307718, "Y"=-0.12533323356430717}, {"X"=-0.9999996829318346, "Y"=-1.0779367755043061e-14}, {"X"=-0.9824361560225743, "Y"=0.1253332335642999}, {"X"=-0.930069338499913, "Y"=0.24868988716485674}, {"X"=-0.8447543509816817, "Y"=0.36812455268467253}, {"X"=-0.7295135194338911, "Y"=0.48175367410171577}, {"X"=-0.5884293077665538, "Y"=0.5877852522924673}, {"X"=-0.42649969451449393, "Y"=0.6845471059286881}, {"X"=-0.24946111695600787, "Y"=0.7705132427757837}, {"X"=-0.0635852549623291, "Y"=0.8443279255020139}, {"X"=0.12454314638835016, "Y"=0.9048270524660212}, {"X"=0.30825954468812783, "Y"=0.9510565162951524}, {"X"=0.48105569493683376, "Y"=0.9822872507286892}, {"X"=0.6368102073656329, "Y"=0.9980267284282712}, {"X"=0.7700054007214531, "Y"=0.9980267284282714}, {"X"=0.8759227688762231, "Y"=0.9822872507286899}, {"X"=0.9508101362587152, "Y"=0.9510565162951536}, {"X"=0.9920145805448566, "Y"=0.9048270524660229}, {"X"=0.9980764137536509, "Y"=0.844327925502016}, {"X"=0.9687808924215855, "Y"=0.7705132427757861}, {"X"=0.9051658249969273, "Y"=0.684547105928691}, {"X"=0.8094848069579983, "Y"=0.5877852522924705}, {"X"=0.6851273860699006, "Y"=0.4817536741017192}, {"X"=0.5364989859650944, "Y"=0.3681245526846762}, {"X"=0.3688648418148406, "Y"=0.2486898871648605}, {"X"=0.18816347674844905, "Y"=0.1253332335643038}, {"X"=0.0007963267107582758, "Y"=7.349118756157295e-15}, {"X"=-0.18659903359769184, "Y"=-0.1253332335643033}, {"X"=-0.36738403011337145, "Y"=-0.24868988716486004}, {"X"=-0.5351542642056617, "Y"=-0.36812455268467575}, {"X"=-0.6839663916912804, "Y"=-0.48175367410171877}, {"X"=-0.8085486687648344, "Y"=-0.58778525229247}, {"X"=-0.9044877061514053, "Y"=-0.6845471059286905}, {"X"=-0.9683848156219029, "Y"=-0.7705132427757859}, {"X"=-0.9979764102178854, "Y"=-0.8443279255020156}, {"X"=-0.9922141929481224, "Y"=-0.9048270524660167}, {"X"=-0.9513022932321045, "Y"=-0.9510565162951535}, {"X"=-0.8766900355135957, "Y"=-0.9822872507286898}, {"X"=-0.7710205962196831, "Y"=-0.9980267284282714}, {"X"=-0.6380373679180417, "Y"=-0.9980267284282712}, {"X"=-0.48245134776907855, "Y"=-0.9822872507286893}, {"X"=-0.3097742481028609, "Y"=-0.9510565162951525}, {"X"=-0.12612324126190735, "Y"=-0.9048270524660215}, {"X"=0.061995744278561214, "Y"=-0.8443279255020141}, {"X"=0.24791849967041305, "Y"=-0.770513242775793}, {"X"=0.4250586186135289, "Y"=-0.6845471059286884}, {"X"=0.5871408240824205, "Y"=-0.5877852522924677}, {"X"=0.7284232731434445, "Y"=-0.4817536741017162}, {"X"=0.8439009646033333, "Y"=-0.368124552684673}, {"X"=0.929483043671546, "Y"=-0.2486898871648572}, {"X"=0.9821377225307711, "Y"=-0.12533323356430037}, {"X"=0.9999996829318346, "Y"=-3.91886975727153e-15}, {"X"=0.9824361560225697, "Y"=0.1253332335643067}, {"X"=0.9300693384999145, "Y"=0.24868988716486337}, {"X"=0.8447543509816838, "Y"=0.3681245526846789}, {"X"=0.7295135194338743, "Y"=0.48175367410172176}, {"X"=0.588429307766557, "Y"=0.5877852522924728}, {"X"=0.4264996945144975, "Y"=0.6845471059286931}, {"X"=0.24946111695598414, "Y"=0.770513242775788}, {"X"=0.06358525496233301, "Y"=0.8443279255020175}, {"X"=-0.12454314638834628, "Y"=0.9048270524660181}, {"X"=-0.30825954468815114, "Y"=0.9510565162951545}, {"X"=-0.4810556949368303, "Y"=0.9822872507286905}, {"X"=-0.6368102073656299, "Y"=0.9980267284282717}, {"X"=-0.7700054007214506, "Y"=0.9980267284282719}, {"X"=-0.8759227688762212, "Y"=0.9822872507286913}, {"X"=-0.9508101362587053, "Y"=0.9510565162951559}, {"X"=-0.992014580544856, "Y"=0.904827052466026}, {"X"=-0.9980764137536511, "Y"=0.8443279255020198}, {"X"=-0.9687808924215935, "Y"=0.7705132427757999}, {"X"=-0.905165824996929, "Y"=0.6845471059286963}, {"X"=-0.8094848069580006, "Y"=0.5877852522924764}, {"X"=-0.6851273860699242, "Y"=0.48175367410172565}, {"X"=-0.5364989859650977, "Y"=0.368124552684683}, {"X"=-0.36886484181484425, "Y"=0.24868988716486765}, {"X"=-0.1881634767484808, "Y"=0.12533323356431106}, {"X"=-0.0007963267107621959, "Y"=1.469947547358777e-14}, {"X"=0.18659903359768798, "Y"=-0.12533323356429601}, {"X"=0.36738403011334136, "Y"=-0.24868988716483917}, {"X"=0.5351542642056584, "Y"=-0.3681245526846689}, {"X"=0.6839663916912776, "Y"=-0.4817536741017123}, {"X"=0.8085486687648153, "Y"=-0.587785252292464}, {"X"=0.9044877061514036, "Y"=-0.6845471059286852}, {"X"=0.9683848156219019, "Y"=-0.7705132427757811}, {"X"=0.9979764102178834, "Y"=-0.8443279255020117}, {"X"=0.992214192948123, "Y"=-0.9048270524660136}, {"X"=0.9513022932321057, "Y"=-0.9510565162951512}, {"X"=0.8766900355136112, "Y"=-0.9822872507286858}, {"X"=0.7710205962196856, "Y"=-0.998026728428271}, {"X"=0.6380373679180447, "Y"=-0.9980267284282718}, {"X"=0.48245134776910686, "Y"=-0.9822872507286906}, {"X"=0.30977424810286464, "Y"=-0.9510565162951549}, {"X"=0.12612324126191124, "Y"=-0.9048270524660246}, {"X"=-0.061995744278528934, "Y"=-0.8443279255020181}, {"X"=-0.24791849967040924, "Y"=-0.7705132427757978}, {"X"=-0.4250586186135254, "Y"=-0.6845471059286937}, {"X"=-0.5871408240823943, "Y"=-0.5877852522924736}, {"X"=-0.7284232731434418, "Y"=-0.48175367410172265}, {"X"=-0.8439009646033313, "Y"=-0.3681245526846798}, {"X"=-0.929483043671534, "Y"=-0.24868988716486432}, {"X"=-0.9821377225307704, "Y"=-0.12533323356430767}, {"X"=-0.9999996829318346, "Y"=-1.1269226474702003e-14}, {"X"=-0.9824361560225757, "Y"=0.1253332335642994}, {"X"=-0.9300693384999159, "Y"=0.2486898871648425}, {"X"=-0.8447543509816858, "Y"=0.3681245526846721}, {"X"=-0.7295135194338964, "Y"=0.4817536741017153}, {"X"=-0.5884293077665601, "Y"=0.5877852522924669}, {"X"=-0.42649969451450104, "Y"=0.6845471059286876}, {"X"=-0.24946111695601544, "Y"=0.7705132427757834}, {"X"=-0.06358525496233693, "Y"=0.8443279255020136}, {"X"=0.12454314638834238, "Y"=0.904827052466015}, {"X"=0.30825954468812033, "Y"=0.9510565162951523}, {"X"=0.48105569493682687, "Y"=0.9822872507286864}, {"X"=0.6368102073656268, "Y"=0.9980267284282712}, {"X"=0.7700054007214481, "Y"=0.9980267284282716}, {"X"=0.8759227688762192, "Y"=0.98228725072869}, {"X"=0.9508101362587128, "Y"=0.9510565162951538}, {"X"=0.9920145805448556, "Y"=0.9048270524660231}, {"X"=0.9980764137536513, "Y"=0.8443279255020162}, {"X"=0.9687808924215875, "Y"=0.7705132427757956}, {"X"=0.9051658249969307, "Y"=0.6845471059286913}, {"X"=0.8094848069580028, "Y"=0.5877852522924824}, {"X"=0.6851273860699063, "Y"=0.48175367410171965}, {"X"=0.536498985965101, "Y"=0.36812455268467664}, {"X"=0.36886484181484785, "Y"=0.24868988716486098}, {"X"=0.18816347674845674, "Y"=0.12533323356430426}, {"X"=0.000796326710766116, "Y"=7.838977475816237e-15}, {"X"=-0.18659903359768412, "Y"=-0.12533323356430282}, {"X"=-0.3673840301133642, "Y"=-0.2486898871648458}, {"X"=-0.535154264205655, "Y"=-0.36812455268467525}, {"X"=-0.6839663916912747, "Y"=-0.4817536741017059}, {"X"=-0.8085486687648298, "Y"=-0.5877852522924696}, {"X"=-0.904487706151402, "Y"=-0.6845471059286902}, {"X"=-0.9683848156219009, "Y"=-0.7705132427757856}, {"X"=-0.997976410217885, "Y"=-0.8443279255020154}, {"X"=-0.9922141929481234, "Y"=-0.9048270524660165}, {"X"=-0.9513022932321069, "Y"=-0.9510565162951533}, {"X"=-0.8766900355135994, "Y"=-0.9822872507286871}, {"X"=-0.7710205962196881, "Y"=-0.9980267284282714}, {"X"=-0.6380373679180477, "Y"=-0.9980267284282713}, {"X"=-0.4824513477690854, "Y"=-0.9822872507286894}, {"X"=-0.30977424810286835, "Y"=-0.9510565162951528}, {"X"=-0.12612324126191513, "Y"=-0.9048270524660217}, {"X"=0.06199574427855339, "Y"=-0.8443279255020144}, {"X"=0.24791849967040544, "Y"=-0.7705132427757934}, {"X"=0.42505861861352184, "Y"=-0.6845471059286887}, {"X"=0.5871408240824142, "Y"=-0.5877852522924796}, {"X"=0.7284232731434391, "Y"=-0.48175367410171666}, {"X"=0.8439009646033292, "Y"=-0.3681245526846735}, {"X"=0.9294830436715431, "Y"=-0.24868988716485768}, {"X"=0.9821377225307696, "Y"=-0.12533323356430087}, {"X"=0.9999996829318346, "Y"=-4.408728476930472e-15}, {"X"=0.9824361560225712, "Y"=0.1253332335643062}, {"X"=0.9300693384999174, "Y"=0.24868988716484913}, {"X"=0.8447543509816879, "Y"=0.3681245526846785}, {"X"=0.7295135194338797, "Y"=0.4817536741017089}, {"X"=0.5884293077665633, "Y"=0.5877852522924725}, {"X"=0.4264996945145046, "Y"=0.6845471059286927}, {"X"=0.24946111695599174, "Y"=0.7705132427757877}, {"X"=0.06358525496234084, "Y"=0.8443279255020173}, {"X"=-0.1245431463883385, "Y"=0.9048270524660179}, {"X"=-0.30825954468814365, "Y"=0.9510565162951544}, {"X"=-0.48105569493682343, "Y"=0.9822872507286877}, {"X"=-0.6368102073656238, "Y"=0.9980267284282717}, {"X"=-0.7700054007214637, "Y"=0.998026728428272}, {"X"=-0.8759227688762175, "Y"=0.9822872507286887}, {"X"=-0.9508101362587116, "Y"=0.9510565162951516}, {"X"=-0.9920145805448586, "Y"=0.9048270524660202}, {"X"=-0.9980764137536515, "Y"=0.8443279255020125}, {"X"=-0.9687808924215884, "Y"=0.7705132427757913}, {"X"=-0.9051658249969202, "Y"=0.6845471059286863}, {"X"=-0.8094848069580052, "Y"=0.5877852522924768}, {"X"=-0.6851273860699092, "Y"=0.4817536741017136}, {"X"=-0.5364989859650804, "Y"=0.36812455268468347}, {"X"=-0.3688648418148515, "Y"=0.24868988716485435}, {"X"=-0.1881634767484606, "Y"=0.12533323356429746}, {"X"=-0.0007963267107416144, "Y"=9.784794780447059e-16}, {"X"=0.1865990335976803, "Y"=-0.12533323356430962}, {"X"=0.3673840301133605, "Y"=-0.24868988716485246}, {"X"=0.5351542642056757, "Y"=-0.36812455268468164}, {"X"=0.6839663916912718, "Y"=-0.4817536741017119}, {"X"=0.8085486687648274, "Y"=-0.5877852522924751}, {"X"=0.9044877061514124, "Y"=-0.6845471059286848}, {"X"=0.9683848156218999, "Y"=-0.7705132427757899}, {"X"=0.9979764102178847, "Y"=-0.8443279255020191}, {"X"=0.9922141929481204, "Y"=-0.9048270524660194}, {"X"=0.9513022932321081, "Y"=-0.9510565162951554}, {"X"=0.8766900355136014, "Y"=-0.9822872507286884}, {"X"=0.7710205962196724, "Y"=-0.9980267284282719}, {"X"=0.6380373679180507, "Y"=-0.9980267284282727}, {"X"=0.48245134776911375, "Y"=-0.9822872507286907}, {"X"=0.3097742481028721, "Y"=-0.951056516295155}, {"X"=0.126123241261919, "Y"=-0.9048270524660248}, {"X"=-0.06199574427852111, "Y"=-0.8443279255020183}, {"X"=-0.24791849967040164, "Y"=-0.770513242775798}, {"X"=-0.4250586186135183, "Y"=-0.684547105928694}, {"X"=-0.587140824082388, "Y"=-0.5877852522924855}, {"X"=-0.7284232731434365, "Y"=-0.4817536741017231}, {"X"=-0.8439009646033271, "Y"=-0.3681245526846935}, {"X"=-0.9294830436715311, "Y"=-0.2486898871648648}, {"X"=-0.9821377225307689, "Y"=-0.12533323356430814}, {"X"=-0.9999996829318346, "Y"=-1.1759085194360944e-14}, {"X"=-0.9824361560225773, "Y"=0.12533323356429893}, {"X"=-0.9300693384999188, "Y"=0.248689887164842}, {"X"=-0.84475435098169, "Y"=0.36812455268467165}, {"X"=-0.7295135194339019, "Y"=0.48175367410170244}, {"X"=-0.5884293077665665, "Y"=0.5877852522924665}, {"X"=-0.42649969451450814, "Y"=0.684547105928677}, {"X"=-0.24946111695602305, "Y"=0.770513242775783}, {"X"=-0.06358525496234475, "Y"=0.8443279255020133}, {"X"=0.12454314638833461, "Y"=0.9048270524660148}, {"X"=0.3082595446881129, "Y"=0.9510565162951521}, {"X"=0.48105569493682, "Y"=0.9822872507286863}, {"X"=0.6368102073656208, "Y"=0.9980267284282712}, {"X"=0.7700054007214431, "Y"=0.9980267284282724}, {"X"=0.8759227688762155, "Y"=0.98228725072869}, {"X"=0.9508101362587105, "Y"=0.9510565162951583}, {"X"=0.9920145805448546, "Y"=0.9048270524660234}, {"X"=0.9980764137536517, "Y"=0.8443279255020165}, {"X"=0.9687808924215894, "Y"=0.7705132427757959}, {"X"=0.905165824996934, "Y"=0.6845471059286916}, {"X"=0.8094848069580075, "Y"=0.5877852522924827}, {"X"=0.6851273860699121, "Y"=0.48175367410172004}, {"X"=0.5364989859651077, "Y"=0.3681245526846903}, {"X"=0.3688648418148552, "Y"=0.24868988716486146}, {"X"=0.18816347674846445, "Y"=0.12533323356431886}, {"X"=0.0007963267107739563, "Y"=8.328836195475178e-15}, {"X"=-0.18659903359767643, "Y"=-0.12533323356430232}, {"X"=-0.36738403011335685, "Y"=-0.24868988716484533}, {"X"=-0.5351542642056484, "Y"=-0.3681245526846748}, {"X"=-0.6839663916912689, "Y"=-0.48175367410170544}, {"X"=-0.8085486687648252, "Y"=-0.5877852522924693}, {"X"=-0.9044877061513986, "Y"=-0.6845471059286794}, {"X"=-0.968384815621899, "Y"=-0.7705132427757853}, {"X"=-0.9979764102178844, "Y"=-0.8443279255020152}, {"X"=-0.9922141929481244, "Y"=-0.9048270524660162}, {"X"=-0.9513022932321094, "Y"=-0.9510565162951532}, {"X"=-0.8766900355136032, "Y"=-0.982287250728687}, {"X"=-0.771020596219693, "Y"=-0.9980267284282713}, {"X"=-0.6380373679180537, "Y"=-0.9980267284282722}, {"X"=-0.48245134776909226, "Y"=-0.9822872507286895}, {"X"=-0.3097742481028758, "Y"=-0.9510565162951573}, {"X"=-0.1261232412619229, "Y"=-0.9048270524660219}, {"X"=0.06199574427854556, "Y"=-0.8443279255020146}, {"X"=0.24791849967039783, "Y"=-0.7705132427757937}, {"X"=0.42505861861351474, "Y"=-0.6845471059286891}, {"X"=0.5871408240824079, "Y"=-0.5877852522924799}, {"X"=0.7284232731434338, "Y"=-0.48175367410171704}, {"X"=0.843900964603325, "Y"=-0.36812455268468713}, {"X"=0.9294830436715402, "Y"=-0.24868988716485815}, {"X"=0.9821377225307681, "Y"=-0.12533323356431544}]
  in  "b":dbl=20.0
  in  "B":dbl=1.0
  in  "A":dbl=1.0
  in  "No. of\nsamples":dbl=1000.0
  in  "fs":dbl=1000.0
  in  "d":dbl=1.57
  in  "a":dbl=30.0
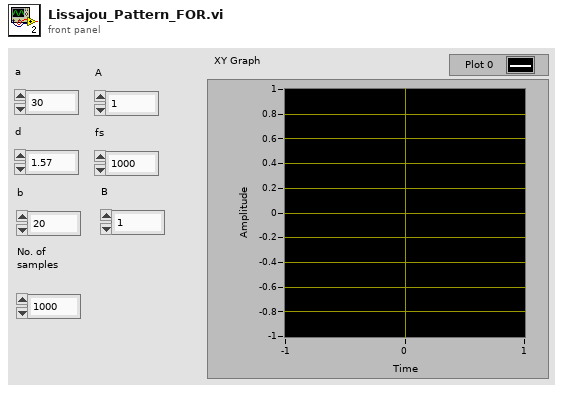
[diagram p1: front panel]
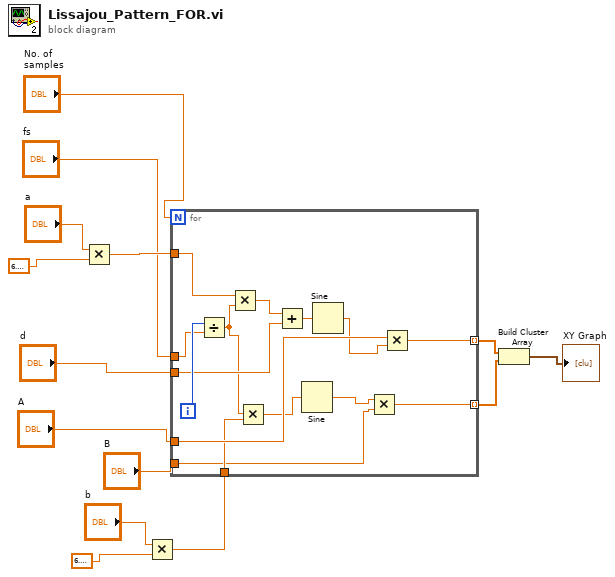
[diagram p0: block diagram]
diagram:
  n1 = Multiply(x="a", y=6.283185307179586) -> (x*y=w12:dbl)
  n2 = Multiply(x="b", y=6.283185307179586) -> (x*y=w6:dbl)
  n3 = for {
    N: "No. of\nsamples" -> [_]
    tunnel: "fs" -> [w28]
    tunnel: w12 -> [w27]
    tunnel: "d" -> [w25]
    tunnel: "A" -> [w24]
    tunnel: w6 -> [w20]
    tunnel: "B" -> [w17]
    tunnel: [w16] -> w2 mode=indexing
    tunnel: [w15] -> w1 mode=indexing
    i -> [w29]
    n4 = Divide(x=w29, y=w28) -> (x/y=w21:dbl)
    n5 = Multiply(x=w27, y=w21) -> (x*y=w26:dbl)
    n6 = Multiply(x=w21, y=w20) -> (x*y=w19:dbl)
    n7 = Add(x=w26, y=w25) -> (x+y=w23:dbl)
    n8 = Sine(x=w19) -> (sin(x)=w18:dbl)
    n9 = Sine(x=w23) -> (sin(x)=w22:dbl)
    n10 = Multiply(x=w18, y=w17) -> (x*y=w15:dbl)
    n11 = Multiply(x=w24, y=w22) -> (x*y=w16:dbl)
  }
  n12 = Build Cluster Array(w2, w1) -> (→"XY Graph":cluster{dbl, dbl}[])
